vi "RegisterBinding.vi"(8 "error in (no error)":errorcluster, 10 "binding parameters":string[](array[string]), 11 "subscriber in":refnum<class "IcmMessageSubscriber.lvclass">) -> (0 "error out":errorcluster, 3 "subscriber out":refnum<class "IcmMessageSubscriber.lvclass">)   [LabVIEW 2017, in "IcmMessageSubscriber.lvclass"]
doc: "Registers a message with particular binding parameters."
uses:
  <vilib>/addons/InsightCM/MessageBus/MessageSubscriber/IcmMessageSubscriber.lvclass
  <vilib>/addons/InsightCM/MessageBus/MessageSubscriber/IcmMessageSubscriber.lvclass/IcmMessageSubscriber.ctl
  C:/Program Files (x86)/National Instruments/LabVIEW 2017/vi.lib/addons/InsightCM/Binaries/LabviewMessageAdapter.dll
  Binaries/LabviewMessageAdapter.dll
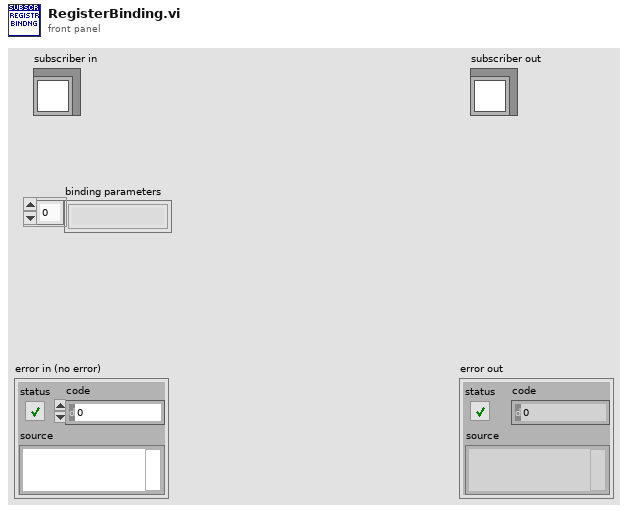
[diagram p1: front panel]
types:
  T1 = typedef "MessageSubscriberDvr.ctl" = refnum<data-value>
  T2 = typedef "MessageSubscriberData.ctl" = cluster{"Subscriber":refnum<k24>}
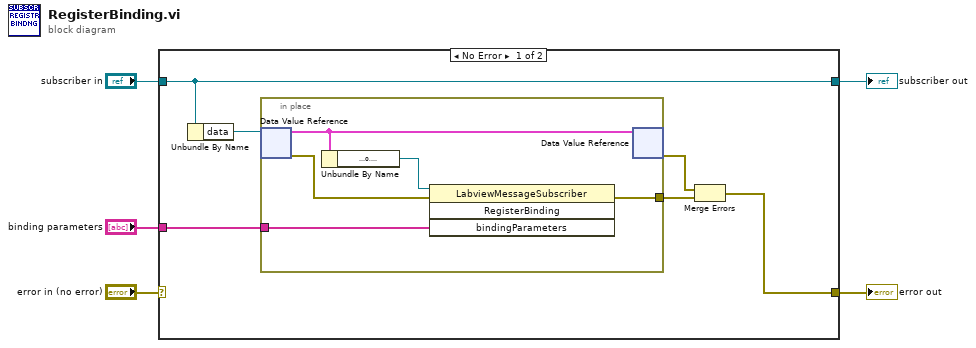
[diagram p0: block diagram]
diagram:
  n1 = case shown="No Error" "error in (no error)" {
    selector: "error in (no error)" -> [_ w18]
    tunnel: [w7 w18] -> w4
    tunnel: "subscriber in" -> [w6 w17]
    tunnel: "binding parameters" -> [w8 _]
    tunnel: [w6 w17] -> w1
    frame No Error {
      n2 = Unbundle By Name(w6) -> ("data"=w11:T1)
      n3 = in-place {
        in-place-border: [w15] -> w9
        in-place-border: w8 -> [w12]
        n4 = in-place-dvr #1(w11) -> (w16:T2, w14:errorcluster)
        n5 = Unbundle By Name(w16) -> ("Subscriber"=w13:refnum<k24>)
        n6 = invoke class="LabviewMessageSubscriber" method="RegisterBinding"(reference=w13, error in=w14, "bindingParameters"=w12) -> (error out=w15:errorcluster)  [unwired: 1 in, 3 out]
        n7 = in-place-dvr #1(w16) -> (w10:errorcluster)  [unwired: 1 out]
      }
      n8 = Merge Errors(w10, w9) -> (w7:errorcluster)
    }
    frame Error {
    }
  }
  "error out" <- w4
  "subscriber out" <- w1
